vi "Pipe Var Intf - Write Variable.vi"(7 "Force Octave cplx output for cplx inputs (True)":bool=TRUE, 8 "error in (no error)":errorcluster, 9 "data in":variant, 10 "variable name":string, 11 "GOLPI ref. in":T1={"pipe handle"={"lv_proc.dll file path"=path "", "process instance handle"=[], "debug mode"=FALSE, "debug data"=[]}, "fast read timeout [ms]"=500, "fast read settle time [ms]"=10, "fast read to multiple [ms]"=1, "max elements per input line"=100, "slow read timeout [ms]"=5000, "stdin double format specifier"="%_16e", "max elements per stdout output column"=100, "console mode bitstream"=FALSE, "bitstream first read timeout [ms]"=1000, "bitstream read timeout [ms]"=50, "struct transfer possible"=FALSE, "matlab mode"=FALSE, "var pipe write timeout [ms]"=5000, "variable pipe mode"=FALSE, "variable pipe buffer size [Bytes]"=10000000, "variable pipe block size [Bytes]"=1000000} {"variable pipe block size [Bytes]" format="%.0p"; "variable pipe buffer size [Bytes]" format="%.0p"}) -> (0 "error out":errorcluster, 3 "GOLPI ref. out":T1={"pipe handle"={"lv_proc.dll file path"=path "", "process instance handle"=[], "debug mode"=FALSE, "debug data"=[]}, "fast read timeout [ms]"=500, "fast read settle time [ms]"=10, "fast read to multiple [ms]"=1, "max elements per input line"=100, "slow read timeout [ms]"=5000, "stdin double format specifier"="", "max elements per stdout output column"=100, "console mode bitstream"=FALSE, "bitstream first read timeout [ms]"=1000, "bitstream read timeout [ms]"=50, "struct transfer possible"=FALSE, "matlab mode"=FALSE, "var pipe write timeout [ms]"=5000, "variable pipe mode"=FALSE, "variable pipe buffer size [Bytes]"=10000000, "variable pipe block size [Bytes]"=1000000} {"variable pipe block size [Bytes]" format="%.0p"; "variable pipe buffer size [Bytes]" format="%.0p"})   [LabVIEW 2020, in "GOLPI library.lvlib"]
doc: "Write matrix to Octave using pipe variable interface."
uses:
  GOLPI library.lvlib
  Public/GOLPI reference Type Def.ctl
  LV Process source distribution/Pipe Handle.ctl
  Pipe Var Intf - Data Type.ctl
  <vilib>/Utility/error.llb/Error Cluster From Error Code.vi
  <vilib>/ErrorRing/Error Ring.xnode
  LV Process source distribution/LV Process library.lvlib
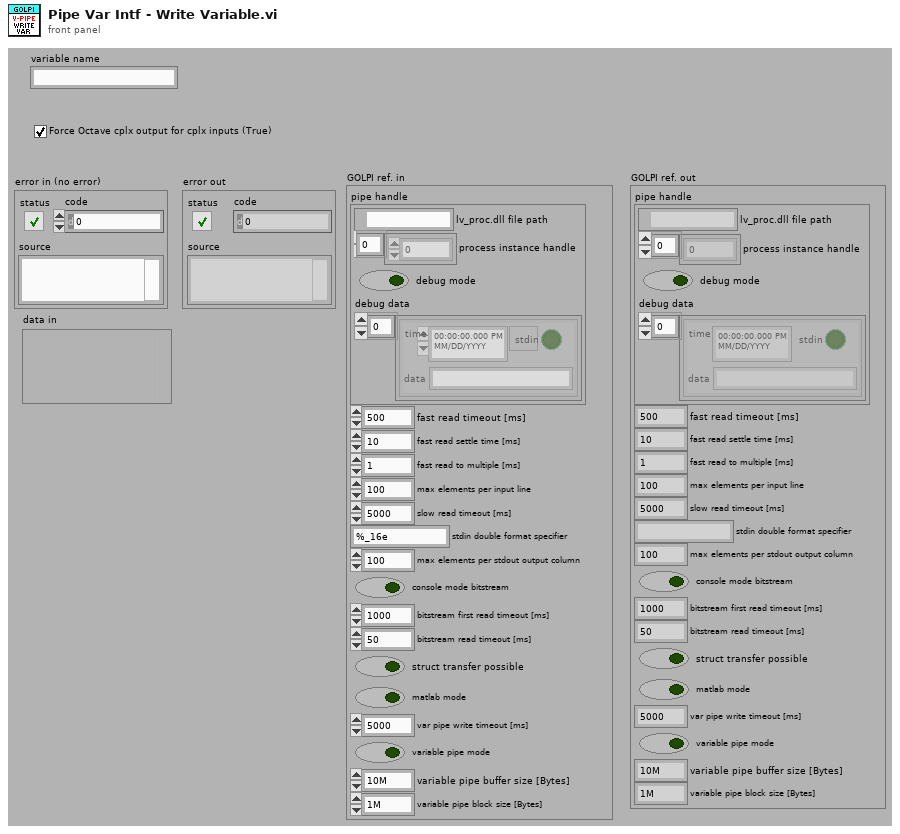
[diagram p1: front panel]
types:
  T1 = typedef "GOLPI library.lvlib/GOLPI reference Type Def.ctl" = cluster{"pipe handle":T2, "fast read timeout [ms]":u32, "fast read settle time [ms]":u32, "fast read to multiple [ms]":u32, "max elements per input line":u32, "slow read timeout [ms]":u32, "stdin double format specifier":string, "max elements per stdout output column":u32, "console mode bitstream":bool, "bitstream first read timeout [ms]":u32, "bitstream read timeout [ms]":u32, "struct transfer possible":bool, "matlab mode":bool, "var pipe write timeout [ms]":u32, "variable pipe mode":bool, "variable pipe buffer size [Bytes]":u32, "variable pipe block size [Bytes]":u32}
  T2 = typedef "LV Process library.lvlib/Pipe Handle.ctl" = cluster{"lv_proc.dll file path":path, "process instance handle":u32[], "debug mode":bool, "debug data":cluster{"time":timestamp, "stdin":bool, "data":string}[]}
  T3 = typedef "NI_Data Type.lvlib/Data Type.ctl" = enum8{"Invalid Type", "Void", "I8", "I16", "I32", "I64", "U8", "U16", "U32", "U64", "Single Float", "Double Float", "Extended Float", "Single Complex", "Double Complex", "Extended Complex", "Enum U8", "Enum U16", "Enum U32", "Enum U64", "Single Float With Unit", "Double Float With Unit", "Extended Float With Unit", "Single Complex with Unit", "Double Complex with Unit", "Extended Complex with Unit", "Boolean", "String", "Path", "Picture", "Tag", "Array", "Cluster", "Variant", "LV Variant", "Waveform", "Timestamp", "Digital Waveform", "Digital Data", "ExpressData", "Refnum", "External Data", "VI", "Poly VI", "LabVIEW Class Instance", "Fixed Point", "Set Collection", "Map Collection"}
  T4 = typedef "GOLPI library.lvlib/Pipe Var Intf - Data Type.ctl" = enum16{"error", "String", "int8", "uint8", "int16", "uint16", "int32", "uint32", "double", "cplx double", "single", "cplx single"}
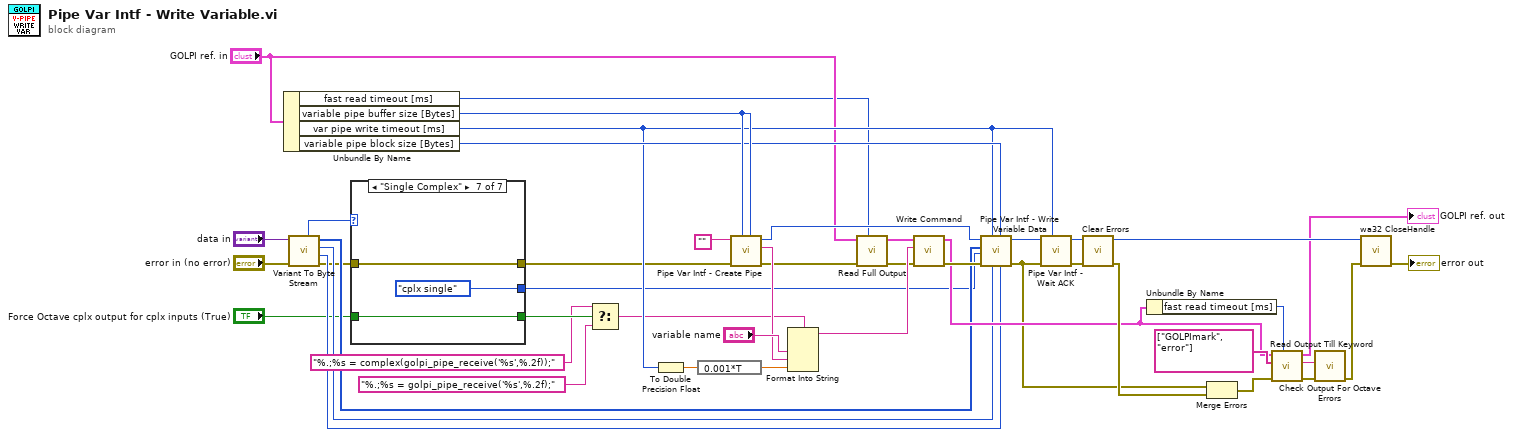
[diagram p0: block diagram]
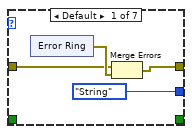
[diagram p2: hidden frame]
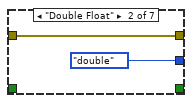
[diagram p3: hidden frame]
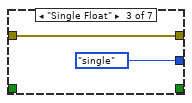
[diagram p4: hidden frame]
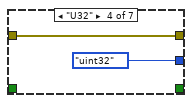
[diagram p5: hidden frame]
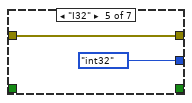
[diagram p6: hidden frame]
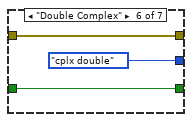
[diagram p7: hidden frame]
diagram:
  n1 = Unbundle By Name("GOLPI ref. in") -> ("fast read timeout [ms]"=w17:u32, "variable pipe buffer size [Bytes]"=w36:u32, "var pipe write timeout [ms]"=w33:u32, "variable pipe block size [Bytes]"=w35:u32)
  n2 = call "Variant To Byte Stream.vi"("error in (no error)"="error in (no error)", "data in"="data in") -> ("error out"=w9:errorcluster, "columns"=w12:i32, "rows"=w13:i32, "binary data out"=w14:u8[], "type"=w11:T3)  [unwired: 5 in]
  n3 = case shown="\"Single Complex\"" w11 {
    tunnel: [Pipe_Var_Intf_-_Data_Type."String" ("data type") Pipe_Var_Intf_-_Data_Type."double" ("data type") Pipe_Var_Intf_-_Data_Type."single" ("data type") Pipe_Var_Intf_-_Data_Type."uint32" ("data type") Pipe_Var_Intf_-_Data_Type."int32" ("data type") Pipe_Var_Intf_-_Data_Type."cplx double" ("data type") Pipe_Var_Intf_-_Data_Type."cplx single" ("data type")] -> w10
    tunnel: [w46 w54 w56 w58 w60 w63 w66] -> w8
    tunnel: w9 -> [w47 w54 w56 w58 w60 w63 w66]
    tunnel: [_ _ _ _ _ w62 w65] -> w4
    tunnel: "Force Octave cplx output for cplx inputs (True)" -> [_ _ _ _ _ w62 w65]
    frame Default {
      n4 = xnode "Error Ring"() -> ("error out"=w48:errorcluster)
      n5 = Merge Errors(w47, w48) -> (w46:errorcluster)
    }
    frame "Double Float" {
    }
    frame "Single Float" {
    }
    frame "U32" {
    }
    frame "I32" {
    }
    frame "Double Complex" {
    }
    frame "Single Complex" {
    }
  }
  n6 = Select(t="%.;%s = complex(golpi_pipe_receive('%s',%.2f));" ("format string"), s=w4, f="%.;%s = golpi_pipe_receive('%s',%.2f);" ("format string")) -> (s? t:f=w1:string)
  n7 = To Double Precision Float(number=w33) -> (double precision float=w32:dbl)
  n8 = expression code="0.001*T"(w32) -> (w34:dbl)
  n9 = call "Pipe Var Intf - Create Pipe.vi"("outBufferSize (256k)"=w36, "inBufferSize (256k)"=w36, "error in (no error)"=w8, "pipe name in (leave empty to generate random name)"="") -> ("error out"=w20:errorcluster, "pipe name out"=w42:string, "pipe handle out"=w40:i32)  [unwired: 5 in]
  n10 = Format Into String(format string=w1, "variable name", w42, w34) -> (resulting string=w41:string)  [unwired: 2 in, 1 out]
  n11 = call "Read Full Output.vi"("timeout [ms]"=w17, "error in"=w20, "GOLPI ref. in"="GOLPI ref. in") -> ("error out"=w21:errorcluster, "GOLPI ref. out"=w18:T1)  [unwired: 5 in, 2 out]
  n12 = call "Write Command.vi"("error in"=w21, "command"=w41, "GOLPI ref. in"=w18) -> ("error out"=w44:errorcluster, "GOLPI ref. out"=w22:T1)  [unwired: 7 in]
  n13 = call "Pipe Var Intf - Write Variable Data.vi"("columns"=w12, "write block size (10k)"=w35, "rows"=w13, "timeout [ms]"=w33, "error in (no error)"=w44, "data type"=w10, "data"=w14, "pipe handle"=w40) -> ("error out"=w6:errorcluster, "pipe handle out"=w37:i32)  [unwired: 2 in]
  n14 = call "Pipe Var Intf - Wait ACK.vi"("timeout [ms]"=w33, "error in (no error)"=w6, "pipe handle"=w37) -> ("error out"=w29:errorcluster, "pipe handle out"=w38:i32)  [unwired: 7 in]
  n15 = call <vilib>:"Clear Errors.vi"("error in (no error)"=w29) -> ("error out"=w24:errorcluster)  [unwired: 5 in, 1 out]
  n16 = Unbundle By Name(w22) -> ("fast read timeout [ms]"=w30:u32)
  n17 = Merge Errors(w6, w24) -> (w7:errorcluster)
  n18 = call "Read Output Till Keyword.vi"("timeout [ms]"=w30, "error in"=w7, "keywords"=string[] ["GOLPImark", "error"], "GOLPI ref. in"=w22) -> ("error out"=w28:errorcluster, "read buffer"=w27:string, "GOLPI ref. out"=→"GOLPI ref. out":T1)  [unwired: 4 in, 1 out]
  n19 = call "Check Output For Octave Errors.vi"("error in"=w28, "read buffer"=w27) -> ("error out"=w23:errorcluster)  [unwired: 9 in]
  n20 = call "wa32 CloseHandle.vi"("error in"=w23, "handle"=w38) -> ("error out"=→"error out":errorcluster)  [unwired: 9 in]
